vi "ReadWriteTest (host).vi"() -> ()   [LabVIEW 2009]
uses:
  <vilib>/rvi/interface/nirviOpenFPGA/nirviOpenFPGA.xnode
  ReadWriteTest (FPGA).vi
  <vilib>/rvi/interface/RandomDataEmulation/nirviRandomDataOpen.vi
  <vilib>/rvi/interface/nirviOpenFPGA/nirviOpenFPGA.ctl
  <vilib>/rvi/interface/nirviOpenFPGA/nirviopenstate.ctl
  <vilib>/picture/picture.llb/imagedata.ctl
  <vilib>/rvi/interface/common/nirviIntfCommonState.ctl
  <vilib>/rvi/interface/common/nirviIntfModes.ctl
  C:/Program Files/National Instruments/LabVIEW 2009/resource/RVI/emulation/niLvFpgaEmulationMode.ctl
  <vilib>/eio/XNode/Errors/EIOXNodeErrorStruct.ctl
  <vilib>/eio/XNode/Errors/EIOXNodeInternalErrorTypes.ctl
  <vilib>/eio/XNode/Errors/EIOXNodeUserErrorTypes.ctl
  <vilib>/XNodeSupport/XNodeRect32.ctl
  <vilib>/XNodeSupport/XNodeInt.ctl
  <vilib>/XNodeSupport/XNodeTerms.ctl
  <vilib>/XNodeSupport/XNodeTerm.ctl
  <vilib>/XNodeSupport/XNodeString.ctl
  <vilib>/XNodeSupport/XNodeVariant.ctl
  <vilib>/XNodeSupport/XNodeBool.ctl
  <vilib>/rvi/interface/nirviReadWriteControl/nirviReadWriteControl.xnode
  <vilib>/userdefined/High Color/nirio_resource_hc.ctl
  <vilib>/XNodeSupport/NI_XNodeSupport.lvlib
panel:
  out "Point Read":cluster{"X":i32, "Y":i32, "Z":i32}
  out "Point Written":cluster{"X":i32, "Y":i32, "Z":i32}
  out "Read Time":u32
  out "Write Time":u32
  out "Count":i32
  out "Matched":cluster{"X":bool, "Y":bool, "Z":bool}
  in  "stop":bool
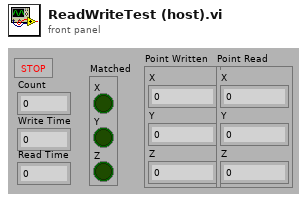
[diagram p1: front panel]
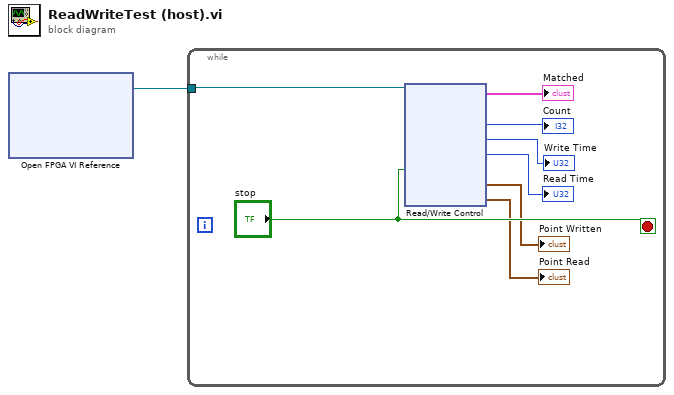
[diagram p0: block diagram]
diagram:
  n1 = xnode "Open FPGA VI Reference"() -> ("FPGA VI Reference Out"=w1:refnum<k20>)  [unwired: 2 in, 1 out]
  n2 = while {
    tunnel: w1 -> [w9]
    stop <- "stop" stop-if-true
    n3 = xnode "Read/Write Control"("FPGA VI Reference In"=w9, "stop"="stop") -> ("Matched"=→"Matched":cluster{"X":bool, "Y":bool, "Z":bool}, "Numeric"=→"Count":i32, "Write Time"=→"Write Time":u32, "Read Time"=→"Read Time":u32, "Point Written"=→"Point Written":cluster{"X":i32, "Y":i32, "Z":i32}, "Point Read"=→"Point Read":cluster{"X":i32, "Y":i32, "Z":i32})  [unwired: 1 in, 2 out]
  }
